vi "XCL Write header.vi"(4 "DC meter idn":string, 6 "AC source idn":string, 7 "Digitizer idn":string, 8 "error in (no error)":errorcluster, 11 "FFmeter settings":T1 {"Measurement properties"."Record length (multiples of period)" format="%#_3p"; "Measurement properties"."Sampling frequency (Hz)" format="%#_3p"; "Measurement properties"."Measurement frequencies (Hz)" format="%#_3p"}) -> (0 "error out":errorcluster, 3 "FFmeter settings out":T1 {"Measurement properties"."Record length (multiples of period)" format="%#_3p"; "Measurement properties"."Sampling frequency (Hz)" format="%#_3p"; "Measurement properties"."Measurement frequencies (Hz)" format="%#_3p"}, 5 "NI_report out":refnum<class "NI_report.lvclass">)   [LabVIEW 2020]
uses:
  GUI/Type definitions/FFmeter settings.ctl
  General AC source/Type definitions/AC Source.ctl
  General AC source/Type definitions/AC Source type.ctl
  General DC meter/Type definitions/DC meter.ctl
  General DC meter/Type definitions/DC meter type.ctl
  Measurement/Type definitions/Measuement properties.ctl
  <vilib>/Utility/NIReport.llb/NI_report.lvclass
  <vilib>/Utility/NIReport.llb/Report Type.ctl
  <vilib>/Utility/NIReport.llb/NI_ReportGenerationCore.lvlib
  external libraries/varilib/varilib.lvlib
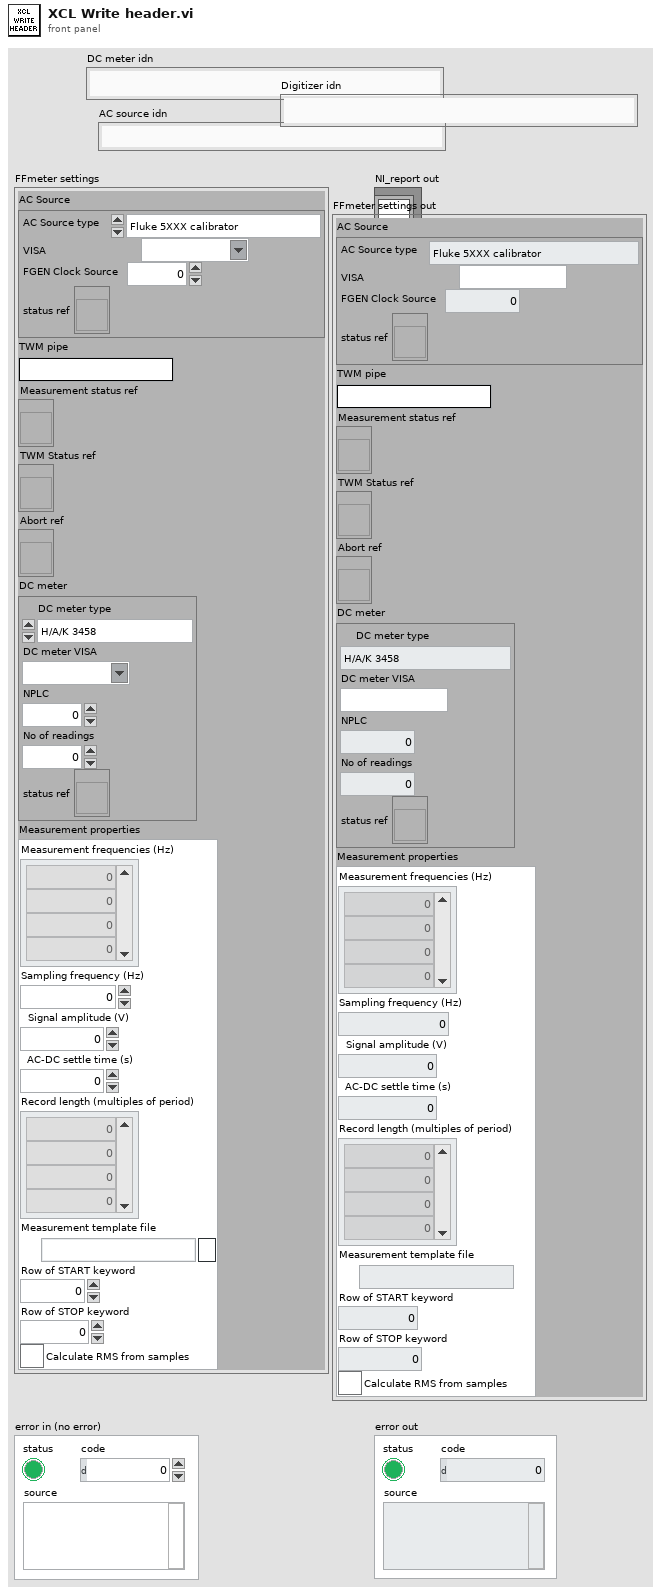
[diagram p1: front panel]
types:
  T1 = typedef "FFmeter settings.ctl" = cluster{"AC Source":T2, "TWM pipe":string, "Measurement status ref":refnum<vi>, "TWM Status ref":refnum<vi>, "Abort ref":refnum<vi>, "DC meter":T4, "Measurement properties":T6}
  T2 = typedef "AC Source.ctl" = cluster{"AC Source type":T3, "VISA":refnum<visa-resource-name>, "Ref. clock (Hz)":dbl, "status ref":refnum<vi>}
  T3 = typedef "AC Source type.ctl" = enum16{"Fluke 5XXX calibrator", "Tektronix AFG3101C", "dummy"}
  T4 = typedef "DC meter.ctl" = cluster{"DC meter type":T5, "DC meter VISA":refnum<visa-resource-name>, "NPLC":i32, "No of readings":i32, "status ref":refnum<vi>}
  T5 = typedef "DC meter type.ctl" = enum16{"H/A/K 3458", "FLuke 8508A", "dummy"}
  T6 = typedef "Measuement properties.ctl" = cluster{"Measurement frequencies (Hz)":dbl[], "Sampling frequency (Hz)":dbl, "Signal amplitude (V)":dbl, "AC-DC settle time (s)":dbl, "Record length (multiples of period)":dbl[], "Measurement template file":path, "Row of START keyword":i32, "Row of STOP keyword":i32, "Calculate RMS from samples":bool}
  T7 = enum16{"maximized", "minimized", "normal", "no change"}
  T8 = typedef "NI_ReportGenerationCore.lvlib/Report Type.ctl" = enum16{"HTML", "Word", "Excel"}
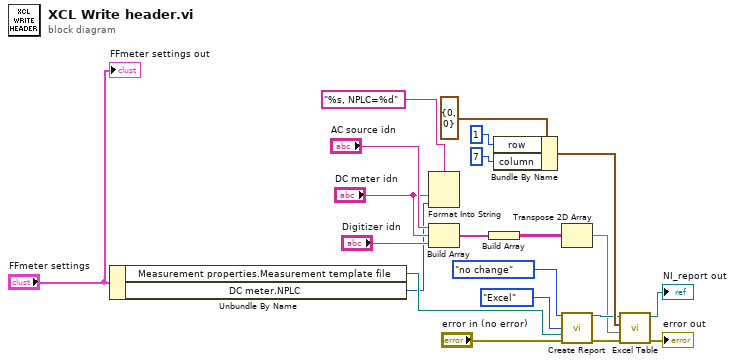
[diagram p0: block diagram]
diagram:
  n1 = Unbundle By Name("FFmeter settings") -> ("Measurement properties.Measurement template file"=w19:path, "DC meter.NPLC"=w1:i32)
  n2 = Format Into String(format string="%s, NPLC=%d", "DC meter idn", w1) -> ()  [unwired: 2 in, 2 out]
  n3 = Build Array("AC source idn", "DC meter idn", "Digitizer idn") -> (w11:string[])
  n4 = Build Array(w11) -> (w6:string[][])
  n5 = Bundle By Name(cluster=cluster{"row":i32, "column":i32} {"row"=0, "column"=0} ("start (0, 0)"), "row"=1, "column"=7) -> (w15:cluster{"row":i32, "column":i32})
  n6 = Transpose 2D Array(2D array=w6) -> (transposed array=w5:string[][])
  n7 = call <vilib>:"Create Report.vi"("window state (normal)"=T7."no change", "report type"=Report_Type."Excel", "template (empty)"=w19, "error in (no error)"="error in (no error)") -> ("report out"=w8:refnum<class "NI_report.lvclass">, "error out"=w10:errorcluster)  [unwired: 10 in]
  n8 = call "Excel Table.vi"("error in (no error)"=w10, "table"=w5, "start (0, 0)"=w15, "report in"=w8) -> ("error out"=→"error out":errorcluster, "report out"=→"NI_report out":refnum<class "NI_report.lvclass">)  [unwired: 6 in]
  "FFmeter settings out" <- "FFmeter settings"
